vi "CursorPosition.vi"(8 "Cursor No.":dbl=1.0, 10 "Cursor":bool=TRUE, 11 "3D Surface Analysis":refnum<k7>(container)) -> (1 "Cursor Z":dbl=1.0, 2 "Cursor Y":dbl=1.0, 3 "Cursor X":dbl=1.0)   [LabVIEW 2018]
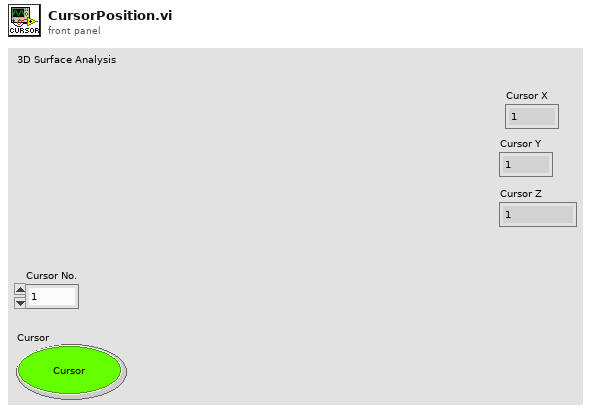
[diagram p1: front panel]
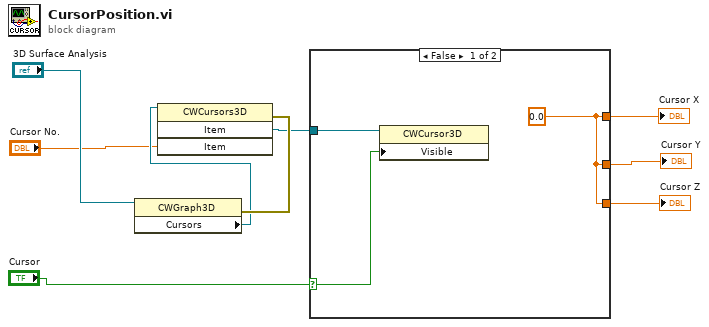
[diagram p0: block diagram]
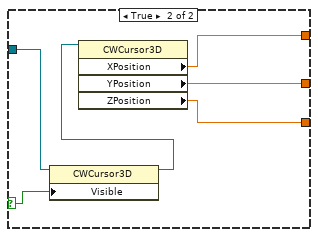
[diagram p2: hidden frame]
diagram:
  n1 = property class="CWGraph3D"(reference="3D Surface Analysis") -> (error out=w9:errorcluster, "Cursors"=w8:refnum<k7>)  [unwired: 1 in, 1 out]
  n2 = invoke class="CWCursors3D" method="Item"(reference=w8, error in=w9, "Item"="Cursor No.") -> ("Item"=w6:refnum<k7>)  [unwired: 1 in, 3 out]
  n3 = case shown="False" "Cursor" {
    selector: "Cursor" -> [w11 w18]
    tunnel: w6 -> [w12 w17]
    tunnel: [w10 w15] -> w3
    tunnel: [w10 w14] -> w2
    tunnel: [w10 w13] -> w1
    frame False {
      w10 = 0.0 ("XPosition")
      n4 = property class="CWCursor3D"(reference=w12, "Visible"=w11) -> ()  [unwired: 1 in, 2 out]
    }
    frame True {
      n5 = property class="CWCursor3D"(reference=w17, "Visible"=w18) -> (reference out=w16:refnum<k7>)  [unwired: 1 in, 1 out]
      n6 = property class="CWCursor3D"(reference=w16) -> ("XPosition"=w15:dbl, "YPosition"=w14:dbl, "ZPosition"=w13:dbl)  [unwired: 1 in, 2 out]
    }
  }
  "Cursor Y" <- w2
  "Cursor X" <- w3
  "Cursor Z" <- w1
